vi "UART Write Bytes.vi"(7 "DataSize":i32, 8 "error in (no error)":errorcluster, 9 "pWriteData":u8[](array[numeric])=array[4097 elements], 10 "Channel":u8, 11 "DevHandle":i32) -> (0 "error out":errorcluster, 1 "pWriteData out":u8[](array[numeric]), 3 "function return":i32)   [LabVIEW 2010, in "usb2uart.lvlib"]
doc: "int WINAPI UART_WriteBytes(int DevHandle,unsigned char Channel,unsigned char *pWriteData,int DataSize);"
uses:
  usb2uart.lvlib
  USB2XXX.dll
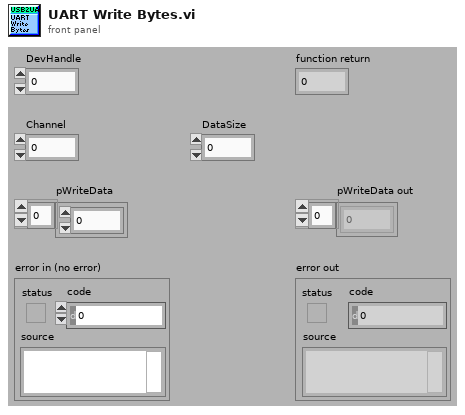
[diagram p1: front panel]
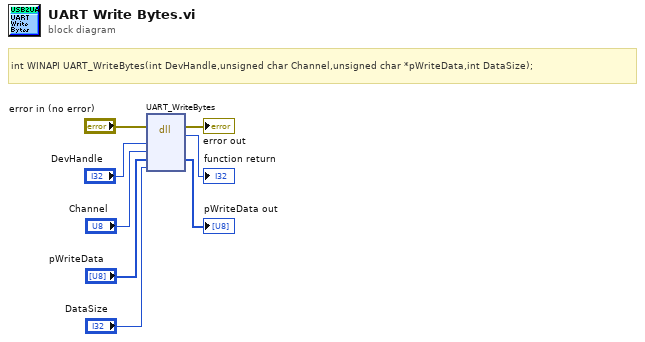
[diagram p0: block diagram]
diagram:
  # "int WINAPI UART_WriteBytes(int DevHandle,unsigned char Channel,unsigned char *pWriteData,int DataSize);"
  n1 = dll-call lib="E:/OtherWork/STM32/USB2XXX_Example/sdk/api/Labview/USB2XXX.*" fn="UART_WriteBytes"(error in="error in (no error)", "DevHandle"="DevHandle", "Channel"="Channel", "pWriteData"="pWriteData", "DataSize"="DataSize") -> (error out=→"error out":errorcluster, →"function return":i32, "pWriteData"=→"pWriteData out":u8[])  [unwired: 5 in, 1 out]
